vi "Initialize.vi"(8 "error in (no error)":errorcluster, 11 "NiPxi6682 in":refnum<class "NiPxi6683H.lvclass">) -> (0 "error out":errorcluster, 3 "NiPxi6682 out":refnum<class "NiPxi6683H.lvclass">)   [LabVIEW 2014, in "SyncPlugins.lvlib" / "NiPxi6683H.lvclass"]
uses:
  NiPxi6683H.lvclass
  NiPxi6682/NiPxi6682.lvclass/NiPxi6682.ctl
  SyncPluginBase/SyncPluginBase.lvclass/SyncPluginBase.ctl
  NiPxi6682/Accessors/Read PgmPPS.vi
  NiPxi6682/Accessors/Read ClkDest.vi
  NiPxi6682/Accessors/Write NiSyncHandle.vi
  SyncPluginBase/Accessors/Write Initiated.vi
  SyncPluginBase/Accessors/Write Locked.vi
  SyncPluginBase/Accessors/Write Run.vi
  NiPxi6682/Accessors/Write SysHandle.vi
  NiPxi6682/Accessors/Write SysRef.vi
  <instrlib>/niSync/niSync.llb/niSync Initialize (IVI).vi
  <instrlib>/niSync/niSync.llb/niSync Set Time Reference (GPS).vi
  <vilib>/nisyscfg/nisyscfg.lvlib
  <resource>/objmgr/niflexriosae.rc
  <resource>/objmgr/nisysapi.rc
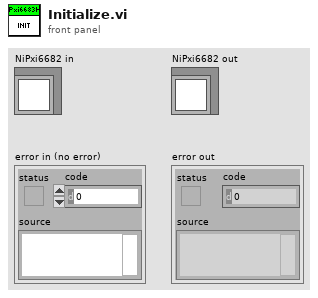
[diagram p1: front panel]
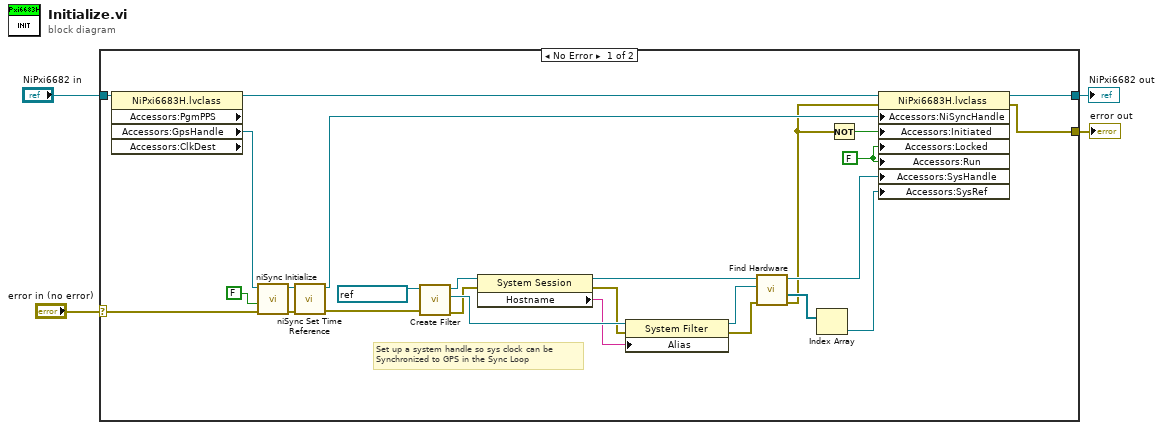
[diagram p0: block diagram]
diagram:
  n1 = case shown="No Error" "error in (no error)" {
    selector: "error in (no error)" -> [w29 w31]
    tunnel: [w24 w32] -> w1
    tunnel: "NiPxi6682 in" -> [w30 w32]
    tunnel: [w5 w31] -> w2
    frame No Error {
      w23 = FALSE ("Locked")
      # "Set up a system handle so sys clock can be\nSynchronized to GPS in the Sync Loop"
      n2 = property class="NiPxi6683H.lvclass" props=["Accessors:PgmPPS", "Accessors:GpsHandle", "Accessors:ClkDest"](reference=w30) -> (reference out=w27:refnum<class "NiPxi6683H.lvclass">, "Accessors:GpsHandle"=w26:refnum<k15>)  [unwired: 1 in, 3 out]
      n3 = call-poly <instrlib>:"niSync Initialize.vi"("error in (no error)"=w29, "reset device (F)"=FALSE, "resource name"=w26) -> ("error out"=w21:errorcluster, "instrument handle out"=w22:refnum<k15>)  [unwired: 7 in]
      n4 = call-poly <instrlib>:"niSync Set Time Reference.vi"("error in (no error)"=w21, "instrument handle"=w22) -> ("error out"=w8:errorcluster, "instrument handle out"=w25:refnum<k15>)  [unwired: 8 in]
      n5 = call <vilib>:"Create Filter.vi"("error in (no error)"=w8, "Session in"=refnum<k21> "localhost") -> ("error out"=w10:errorcluster, "Filter out"=w20:refnum<k20>, "Session out"=w18:refnum<k21>)  [unwired: 7 in]
      n6 = property class="System Session"(reference=w18, error in=w10) -> (reference out=w16:refnum<k21>, error out=w9:errorcluster, "Hostname"=w17:string)
      n7 = property class="System Filter"(reference=w20, error in=w9, "Alias"=w17) -> (reference out=w15:refnum<k20>, error out=w14:errorcluster)
      n8 = call <vilib>:"Find Hardware.vi"("error in (no error)"=w14, "Filter in"=w15, "Session in"=w16) -> ("error out"=w6:errorcluster, "Resources out"=w13:refnum<k20>[], "Session out"=w11:refnum<k21>)  [unwired: 5 in, 1 out]
      n9 = Index Array(array=w13) -> (element=w12:refnum<k20>)  [unwired: 1 in]
      n10 = Not(x=w6) -> (.not. x?=w7:bool)
      n11 = property class="NiPxi6683H.lvclass"(reference=w27, error in=w6, "Accessors:NiSyncHandle"=w25, "Accessors:Initiated"=w7, "Accessors:Locked"=w23, "Accessors:Run"=w23, "Accessors:SysHandle"=w11, "Accessors:SysRef"=w12) -> (reference out=w24:refnum<class "NiPxi6683H.lvclass">, error out=w5:errorcluster)
    }
    frame Error {
    }
  }
  "error out" <- w2
  "NiPxi6682 out" <- w1
